vi "Test Write and Read Data.vi"() -> ()   [LabVIEW 2019, in "LV-Data.PGSQL.lvclass"]
uses:
  LV-Data.PGSQL.lvclass
  API/Write Variable (one-row).vi
  API/Read Variable (double).vi
panel:
  in  "single (F = multirows)":bool
  out "Read Cluster":T1
  out "Write Cluster":T2
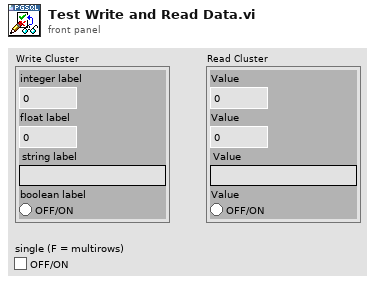
[diagram p1: front panel]
types:
  T1 = cluster{"Value":dbl, "Value":dbl, "Value":string, "Value":bool}
  T2 = cluster{"integer label":i32, "float label":dbl, "string label":string, "boolean label":bool}
  T3 = cluster{"integer label":i32, "float label":dbl, "string label":string, "boolean label":bool, "timestamp label":timestamp}[]
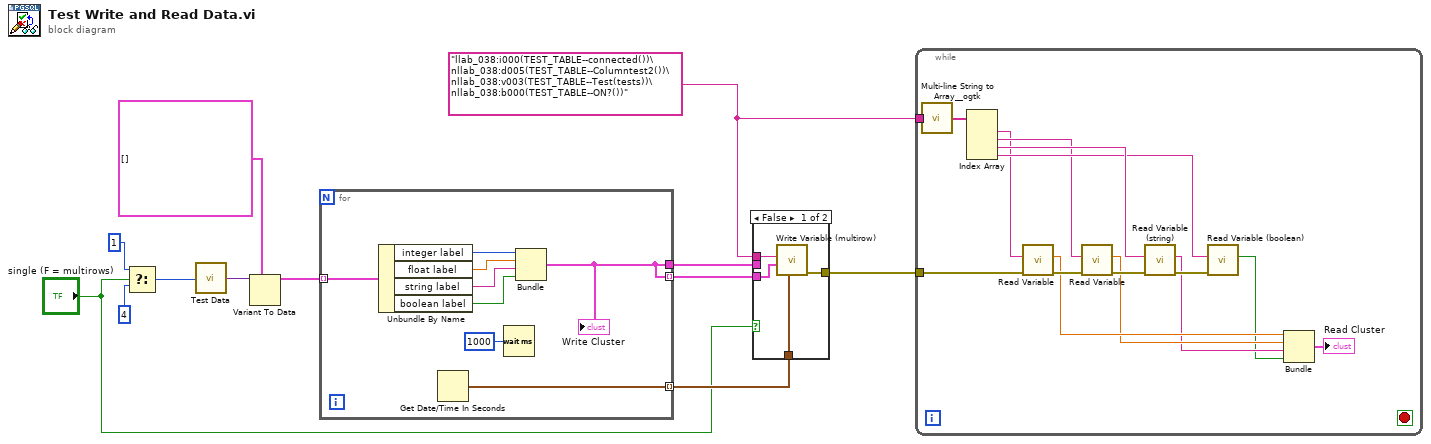
[diagram p0: block diagram]
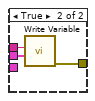
[diagram p2: hidden frame]
diagram:
  w8 = "llab_038:i000(TEST_TABLE--connected())\nllab_038:d005(TEST_TABLE--Columntest2())\nllab_038:v003(TEST_TABLE--Test(tests))\nllab_038:b000(TEST_TABLE--ON?())" ("variable")
  n1 = Select(t=1, s="single (F = multirows)", f=4 ("Size")) -> (s? t:f=w3:i32)
  n2 = call "Test Data.vi"("Size"=w3) -> ("Data"=w11:variant)
  n3 = Variant To Data(type=T3 [] ("cluster"), Variant=w11) -> (data=w10:T3)  [unwired: 1 in, 1 out]
  n4 = for {
    tunnel: w10 -> [w16] mode=indexing
    tunnel: [w15] -> w9
    tunnel: [w15] -> w6 mode=indexing
    tunnel: [w14] -> w7 mode=indexing
    n5 = Unbundle By Name(w16) -> ("integer label"=w20:i32, "float label"=w19:dbl, "string label"=w18:string, "boolean label"=w17:bool)
    n6 = Get Date/Time In Seconds() -> (seconds since 1Jan1904=w14:timestamp)
    n7 = Wait (ms)(milliseconds to wait=u32 1000) -> ()  [unwired: 1 out]
    n8 = Bundle("integer label"=w20, "float label"=w19, "string label"=w18, "boolean label"=w17) -> (w15:T2)  [unwired: 1 in]
    "Write Cluster" <- w15
  }
  n9 = case shown="False" "single (F = multirows)" {
    tunnel: w9 -> [_ w27]
    tunnel: w8 -> [w21 w26]
    tunnel: [w24 w25] -> w1
    tunnel: w7 -> [w23 _]
    tunnel: w6 -> [w22 _]
    frame False {
      n10 = call "Write Variable (multirow).vi"("Time Stamps"=w23, "Data"=w22, "variable"=w21) -> ("error out"=w24:errorcluster)  [unwired: 5 in, 3 out]
    }
    frame True {
      n11 = call-poly "Write Variable.vi"("Data"=w27, "variable"=w26) -> ("error out"=w25:errorcluster)  [unwired: 6 in, 3 out]
    }
  }
  n12 = while {
    tunnel: w8 -> [w30]
    tunnel: w1 -> [w29]
    stop <- w28 stop-if-true
    n13 = call <userlib>:"Multi-line String to Array__ogtk.vi"("string"=w30) -> ("lines"=w40:string[])
    n14 = Index Array(array=w40) -> (element #1=w36:string, element #2=w37:string, element #3=w39:string, element #4=w38:string)  [unwired: 4 in]
    n15 = call-poly "Read Variable.vi"("error in (no error)"=w29, "PG path"=w36) -> ("error out"=w43:errorcluster, "Value"=w35:dbl)  [unwired: 4 in, 4 out]
    n16 = call-poly "Read Variable.vi"("error in (no error)"=w43, "PG path"=w37) -> ("error out"=w42:errorcluster, "Value"=w34:dbl)  [unwired: 4 in, 4 out]
    n17 = call "Read Variable (string).vi"("error in (no error)"=w42, "PG path"=w39) -> ("error out"=w41:errorcluster, "Value"=w33:string)  [unwired: 4 in, 4 out]
    n18 = call "Read Variable (boolean).vi"("error in (no error)"=w41, "PG path"=w38) -> ("Value"=w32:bool)  [unwired: 4 in, 5 out]
    n19 = Bundle("Value"=w35, "Value"=w34, "Value"=w33, "Value"=w32) -> (→"Read Cluster":T1)  [unwired: 1 in]
  }
